vi "Filter String_Arrow Key Handler_ACAF.vi"(8 "error in (no error)":errorcluster, 9 "Done Ref":refnum<vi>, 10 "Filter String Ref":refnum<vi>, 11 "Tree Ref Array":refnum<vi>[](array[refnum])) -> (0 "error out":errorcluster)   [LabVIEW 2023]
doc: "Call the filter and tree arrow handler. \n\nDown arrow or tab from filter goes to tree's first selectable item. Up arrow from filter goes to tree's last selectable item\n\nFilter arrows cycle on tree elements. Shift-tab from tree goes to filter"
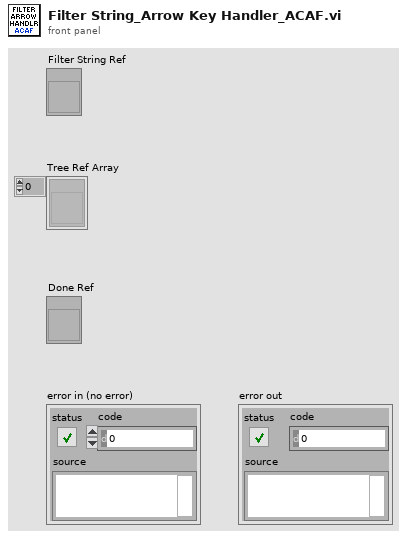
[diagram p1: front panel]
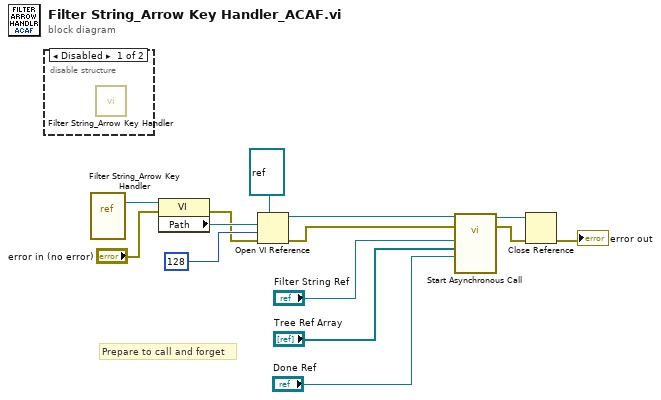
[diagram p0: block diagram]
diagram:
  # "Prepare to call and forget"
  n1 = disable-structure shown="Disabled" {
    frame Disabled {
      n2 = call "Filter String_Arrow Key Handler.vi"() -> ()  [unwired: 12 in]
    }
    frame Enabled {
    }
  }
  n3 = vi-ref "Filter String_Arrow Key Handler.vi"() -> (w14:refnum<vi>)
  n4 = property class="VI"(reference=w14, error in="error in (no error)") -> (error out=w4:errorcluster, "Path"=w10:path)  [unwired: 1 out]
  n5 = Open VI Reference(type specifier VI Refnum (for type only)=refnum<vi> refnum, vi path=w10, options=128, error in (no error)=w4) -> (vi reference=w5:refnum<vi>, error out=w9:errorcluster)  [unwired: 2 in]
  n6 = call-by-ref "Start Asynchronous Call"(reference=w5, error in=w9, "Done Ref"="Done Ref", "Tree Ref Array"="Tree Ref Array", "Filter String Ref"="Filter String Ref") -> (reference out=w8:refnum<vi>, error out=w7:errorcluster)  [unwired: 9 in]
  n7 = Close Reference(reference=w8, error in (no error)=w7) -> (error out=→"error out":errorcluster)
